vi "Read Thermocouple Channel.vi"(8 "error in":errorcluster, 11 "thermocouple channel in":refnum<class "Thermocouple Channel.lvclass">) -> (0 "error out":errorcluster, 1 "default value":dbl, 2 "name":string, 3 "thermocouple channel out":refnum<class "Thermocouple Channel.lvclass">, 4 "index":i32, 5 "thermocouple channel settings":T1)   [LabVIEW 2017, in "Scan Engine Scripting.lvlib" / "Thermocouple Channel.lvclass"]
doc: "Reads the name, thermocouple settings, index and default value of a channel."
uses:
  Thermocouple Channel.lvclass
  C:/dev/niveristand-scan-engine-ethercat-custom-device/Custom Device Source/Scripting/Modules/Channel Classes/Analog Channel/Analog Channel.lvclass
  Thermocouple Channel Settings.ctl
  Thermocouple Type.ctl
  Measurement Units.ctl
  Analog Channel/Analog Channel.lvclass
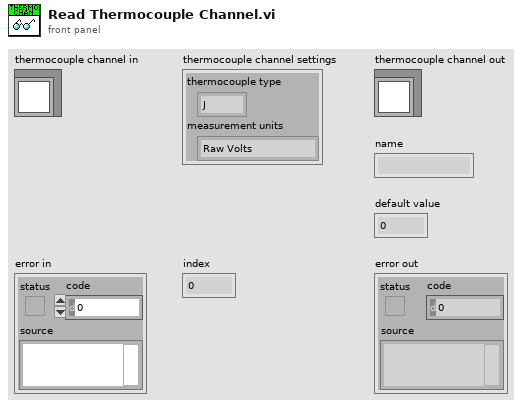
[diagram p1: front panel]
types:
  T1 = typedef "Scan Engine Scripting.lvlib/Thermocouple Channel.lvclass/Thermocouple Channel Settings.ctl" = cluster{"thermocouple type":T2, "measurement units":T3}
  T2 = typedef "Scan Engine Scripting.lvlib/Thermocouple Channel.lvclass/Thermocouple Type.ctl" = enum16{"J", "K", "T", "E", "R", "S", "N", "B"}
  T3 = typedef "Scan Engine Scripting.lvlib/Thermocouple Channel.lvclass/Measurement Units.ctl" = enum16{"Raw Volts", "Degrees Kelvin", "Degrees Celsius", "Degrees Fahrenheit", "Degrees Rankine"}
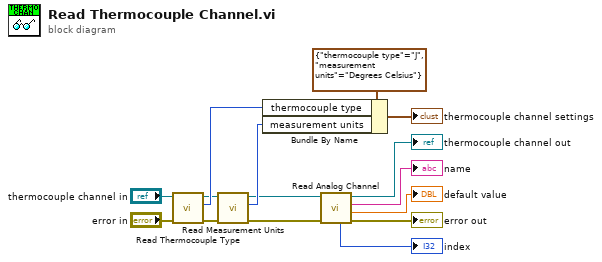
[diagram p0: block diagram]
diagram:
  n1 = call-dynamic "Read Thermocouple Type.vi"("error in"="error in", "thermocouple channel in"="thermocouple channel in") -> ("error out"=w8:errorcluster, "thermocouple type"=w13:T2, "thermocouple channel out"=w11:refnum<class "Thermocouple Channel.lvclass">)  [unwired: 7 in]
  n2 = call-dynamic "Read Measurement Units.vi"("error in"=w8, "thermocouple channel in"=w11) -> ("error out"=w7:errorcluster, "measurement units"=w12:T3, "thermocouple channel out"=w6:refnum<class "Thermocouple Channel.lvclass">)  [unwired: 7 in]
  n3 = Bundle By Name(cluster=T1 {"thermocouple type"=enum."J", "measurement units"=enum."Degrees Celsius"} ("thermocouple channel settings"), "thermocouple type"=w13, "measurement units"=w12) -> (→"thermocouple channel settings":T1)
  n4 = call "Read Analog Channel.vi"("error in"=w7, "analog channel in"=w6) -> ("error out"=→"error out":errorcluster, "default value"=→"default value":dbl, "name"=→"name":string, "analog channel out"=→"thermocouple channel out":refnum<class "Thermocouple Channel.lvclass">, "index"=→"index":i32)  [unwired: 5 in]
